vi "komparator.vi"(1 "Docelowa":dbl, 2 "Aktualna":dbl) -> (0 "Output":string)   [LabVIEW 2024]
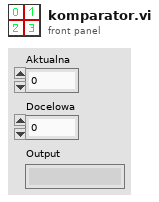
[diagram p1: front panel]
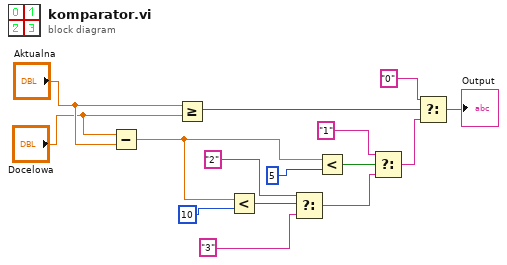
[diagram p0: block diagram]
diagram:
  n1 = Subtract(x="Docelowa", y="Aktualna") -> (x-y=w5:dbl)
  n2 = Greater Or Equal?(x="Aktualna", y="Docelowa") -> (x >= y?=w2:bool)
  n3 = Less?(x=w5, y=10) -> (x < y?=w9:bool)
  n4 = Select(t="2", s=w9, f="3") -> (s? t:f=w7:string)
  n5 = Less?(x=w5, y=5) -> (x < y?=w12:bool)
  n6 = Select(t="1", s=w12, f=w7) -> (s? t:f=w6:string)
  n7 = Select(t="0", s=w2, f=w6) -> (s? t:f=→"Output":string)
